vi "Strings to Connections.vi"(11 "connection strings":string[](array[string])) -> (3 "connection list":T1[](array[typedef]))   [LabVIEW 2017, in "Switch Scripting.lvlib"]
uses:
  Switch Scripting.lvlib
  Routing Channel/Connection.ctl
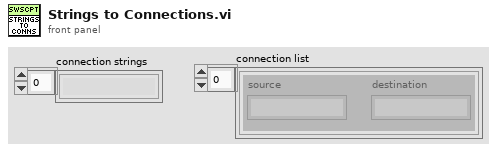
[diagram p1: front panel]
types:
  T1 = typedef "Switch Scripting.lvlib/Connection.ctl" = cluster{"source":string, "destination":string}
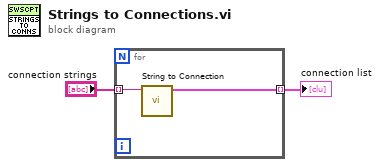
[diagram p0: block diagram]
diagram:
  n1 = for {
    tunnel: [w4] -> w1 mode=indexing
    tunnel: "connection strings" -> [w3] mode=indexing
    n2 = call "String to Connection.vi"("String"=w3) -> ("Connection"=w4:T1)  [unwired: 10 in]
  }
  "connection list" <- w1
